vi "Connect to Server.vi"(4 "timeout (2000 ms)":i32=2000, 5 "Connect Flags":T3={"Reserved"=FALSE, "Clean Session"=TRUE, "Will Flag"=FALSE, "Will QoS 1"=FALSE, "Will QoS 2"=FALSE, "Will Retain"=FALSE, "Password Flag"=FALSE, "User Name Flag"=FALSE}, 6 "Keep Alive (s)":u16, 7 "Payload":T2, 8 "error in (no error)":errorcluster, 11 "Client in":refnum<class "Client.lvclass">) -> (0 "error out":errorcluster, 1 "timed out":bool, 2 "Return Code":T1=enum."Server Unavailable", 3 "Client out":refnum<class "Client.lvclass">)   [LabVIEW 2013, in "MQTT Client.lvlib" / "Client.lvclass"]
uses:
  Client.lvclass
  <vilib>/LabVIEW Open Source Project/MQTT Control Packets/Control Packets/CONNECT/ConnectFlags -- cluster.ctl
  <vilib>/LabVIEW Open Source Project/MQTT Control Packets/Control Packets/CONNACK/Connect Return Code -- enum.ctl
  <vilib>/LabVIEW Open Source Project/MQTT Control Packets/Control Packets/CONNACK/CONNACK.lvclass
  Session.Client/Session.Client.lvclass
  MQTT_Base/Base Class/MQTT_Base.lvclass/MQTT_Base.ctl
  Client.lvclass/Client.ctl
  <vilib>/LabVIEW Open Source Project/MQTT Control Packets/Control Packets/ControlPacket/ControlPacket.lvclass
  <vilib>/LabVIEW Open Source Project/MQTT Control Packets/Control Packets/CONNECT/CONNECT.lvclass
  MQTT_Base/Session/Session.lvclass
  MQTT_Base/Base Class/MQTT_Base.lvclass
  MQTT_Connection/Connection/Connection.lvclass
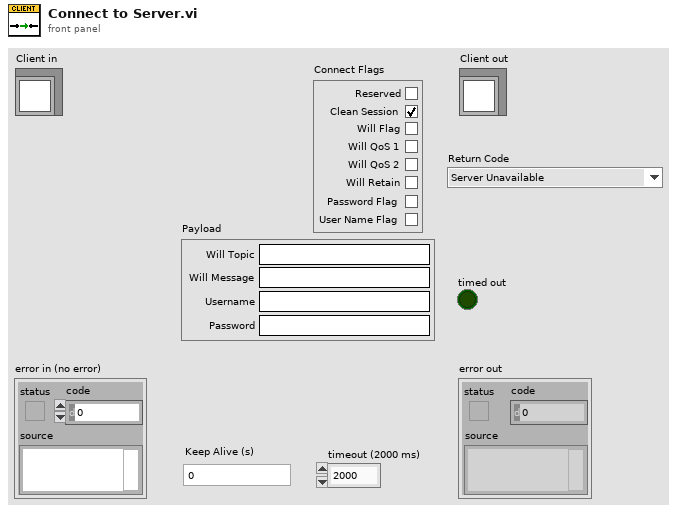
[diagram p1: front panel]
types:
  T1 = typedef "MQTT_Control_Packets.lvlib/CONNACK.lvclass/Connect Return Code -- enum.ctl" = enum16{"Connection accepted", "Unacceptable protocol version", "Identifier Rejected", "Server Unavailable", "Bad Username or Password", "Not Authorized"}
  T2 = cluster{"Will Topic":string, "Will Message":string, "Username":string, "Password":string}
  T3 = typedef "MQTT_Control_Packets.lvlib/CONNECT.lvclass/ConnectFlags -- cluster.ctl" = cluster{"Reserved":bool, "Clean Session":bool, "Will Flag":bool, "Will QoS 1":bool, "Will QoS 2":bool, "Will Retain":bool, "Password Flag":bool, "User Name Flag":bool}
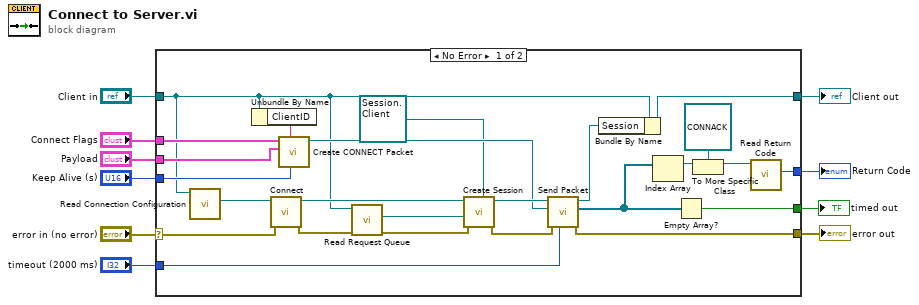
[diagram p0: block diagram]
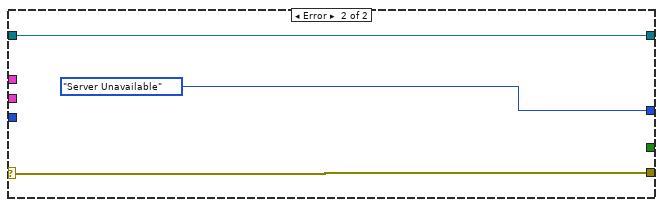
[diagram p2: hidden frame]
diagram:
  n1 = case shown="No Error" "error in (no error)" {
    selector: "error in (no error)" -> [w15 w38]
    tunnel: [w17 w38] -> w9
    tunnel: [w35 w37] -> w7
    tunnel: "Client in" -> [w12 w37]
    tunnel: "Connect Flags" -> [w34 _]
    tunnel: "Payload" -> [w33 _]
    tunnel: "Keep Alive (s)" -> [w32 _]
    tunnel: [w21 _] -> w3
    tunnel: "timeout (2000 ms)" -> [w27 _]
    tunnel: [w23 Connect_Return_Code_--_enum."Server Unavailable" ("Return Code")] -> w1
    frame No Error {
      n2 = call "Read Connection Configuration.vi"("MQTT_Base in"=w12) -> ("Connection Configuration"=w11:refnum<class "Connection.lvclass">)  [unwired: 8 in, 2 out]
      n3 = Unbundle By Name(w12) -> ("ClientID"=w31:string)
      n4 = call "Connect.vi"("error in (no error)"=w15, "Connection in"=w11) -> ("error out"=w14:errorcluster, "Connection out"=w13:refnum<class "Connection.lvclass">)  [unwired: 8 in]
      n5 = call <vilib>:"Create CONNECT Packet.vi"("Keep Alive (s)"=w32, "Client ID (empty: generate new)"=w31, "Payload"=w33, "Connect Flags"=w34) -> ("CONNECT"=w28:refnum<class "CONNECT.lvclass">)  [unwired: 5 in, 2 out]
      n6 = call "Read Request Queue.vi"("error in (no error)"=w14, "MQTT_Base in"=w12) -> ("error out"=w20:errorcluster, "Request"=w30:refnum<queue>)  [unwired: 7 in, 1 out]
      n7 = call "Create Session.vi"("Session in"=refnum<class "Session.Client.lvclass"> refnum ("MQTT Client.lvlib:Session.Client.lvclass"), "error in (no error)"=w20, "Request"=w30, "Connection"=w13) -> ("error out"=w16:errorcluster, "Session"=w29:refnum<class "Session.Client.lvclass">)  [unwired: 6 in]
      n8 = call "Send Packet.vi"("timeout (0ms : no ack)"=w27, "error in (no error)"=w16, "Packet"=w28, "Session in"=w29) -> ("error out"=w17:errorcluster, "Response"=w22:refnum<class "ControlPacket.lvclass">[], "Session out"=w19:refnum<class "Session.Client.lvclass">)  [unwired: 4 in, 1 out]
      n9 = Bundle By Name(cluster=w12, "Session"=w19) -> (w35:refnum<class "Client.lvclass">)
      n10 = Index Array(array=w22) -> (element=w26:refnum<class "ControlPacket.lvclass">)  [unwired: 1 in]
      n11 = Empty Array?(array=w22) -> (empty?=w21:bool)
      n12 = To More Specific Class(target class=refnum<class "CONNACK.lvclass"> refnum ("CONNACK.lvclass"), reference=w26) -> (specific class reference=w24:refnum<class "CONNACK.lvclass">)  [unwired: 1 in, 1 out]
      n13 = call <vilib>:"Read Return Code.vi"("CONNACK in"=w24) -> ("Return Code"=w23:T1)  [unwired: 8 in, 2 out]
    }
    frame Error {
    }
  }
  "error out" <- w9
  "Client out" <- w7
  "timed out" <- w3
  "Return Code" <- w1
